vi "PIM Update Test Results.vi"(5 "PIM Test Results":T11={"Measurement Cycles"=0, "Calibration State"=FALSE, "Data"=[], "PIM Test Parameters"={"Stimulus"={"C1 Pwr dBm"=43.0, "C2 Pwr dBm"=43.0, "Power Units"=enum."dBm", "Meas Type"=enum."Time", "C1 Freq MHz"=0.0, "C2 Freq MHz"=0.0, "Swept Freq Step"=0}, "Measure"={"IM Order"=0, "Direction"=0, "Averaging"=2, "ALC ON?"=TRUE, "Peak Hold?"=TRUE, "Peak last N"=0, "Ref Level dBm"=-100.0, "Ref Units"=enum."dBm", "Num Samples"=0, "Sample units"=enum."Sample(s)", "Update Rate (s)"=0.0, "DUT PORT"=enum."Port 1", "Percent (%)"=100}, "Display"={"Power Scale"={"yRange_min"=-160, "yRange_max"=-60}, "xRange_span"=1}}, "Peak IM Level"=0.0, "Instrument String"="", "Instrument Used"={"ixInstrument"=0, "sxInstrumentId"="", "sDriverId"="", "sDriverType"="", "sSerialNumber"="", "tLastCalibration"=timestamp(0 s since 1904-01-01), "tCalibrationDue"=timestamp(0 s since 1904-01-01), "sConfiguration"=""}} {"PIM Test Parameters"."Stimulus"."Swept Freq Step" items=[".2", ".4", "1.0", "2.0"]; "PIM Test Parameters"."Measure"."Averaging" items=["None", "Minimum", "Normal", "High", "Maximum"]; "PIM Test Parameters"."Measure"."Direction" items=["Reverse", "Forward", "Auxiliary"]; "PIM Test Parameters"."Measure"."IM Order" items=["3rd", "5th", "7th", "9th", "11th", "13th", "15th", "17th", "19th", "21st", "23rd", "25th", "27th", "29th", "31st", "33rd"]}, 7 "Increment Cycles?":bool, 9 "PIM Test Parameters":T1={"Stimulus"={"C1 Pwr dBm"=0.0, "C2 Pwr dBm"=0.0, "Power Units"=enum."dBm", "Meas Type"=enum."Time", "C1 Freq MHz"=0.0, "C2 Freq MHz"=0.0, "Swept Freq Step"=0}, "Measure"={"IM Order"=0, "Direction"=0, "Averaging"=1, "ALC ON?"=TRUE, "Peak Hold?"=TRUE, "Peak last N"=1, "Ref Level dBm"=-100.0, "Ref Units"=enum."dBm", "Num Samples"=1, "Sample units"=enum."Sample(s)", "Update Rate (s)"=0.0, "DUT PORT"=enum."Port 1", "Percent (%)"=100}, "Display"={"Power Scale"={"yRange_min"=0, "yRange_max"=0}, "xRange_span"=5}} {"Stimulus"."Swept Freq Step" items=[".2", ".4", "1.0", "2.0"]; "Measure"."Averaging" items=["None", "Minimum", "Normal", "High", "Maximum"]; "Measure"."Direction" items=["Reverse", "Forward", "Auxiliary"]; "Measure"."IM Order" items=["3rd", "5th", "7th", "9th", "11th", "13th", "15th", "17th", "19th", "21st", "23rd", "25th", "27th", "29th", "31st", "33rd"]}, 10 "Passed?":bool, 12 "Start Time":dbl, 13 "Discard Measurement":bool, 14 "Measurement Results":T13 {"IMPower_dBc(s)" format="%.2f"; "TxFreqs" format="%.2f"; "IMFreq(s)" format="%.2f"; "IMPower(s)" format="%.2f"; "TxPower" format="%.2f"}) -> (6 "Updated Test Results":T11={"Measurement Cycles"=0, "Calibration State"=FALSE, "Data"=[], "PIM Test Parameters"={"Stimulus"={"C1 Pwr dBm"=43.0, "C2 Pwr dBm"=43.0, "Power Units"=enum."dBm", "Meas Type"=enum."Time", "C1 Freq MHz"=0.0, "C2 Freq MHz"=0.0, "Swept Freq Step"=0}, "Measure"={"IM Order"=0, "Direction"=0, "Averaging"=2, "ALC ON?"=TRUE, "Peak Hold?"=TRUE, "Peak last N"=0, "Ref Level dBm"=-100.0, "Ref Units"=enum."dBm", "Num Samples"=0, "Sample units"=enum."Sample(s)", "Update Rate (s)"=0.0, "DUT PORT"=enum."Port 1", "Percent (%)"=100}, "Display"={"Power Scale"={"yRange_min"=-160, "yRange_max"=-60}, "xRange_span"=1}}, "Peak IM Level"=0.0, "Instrument String"="", "Instrument Used"={"ixInstrument"=0, "sxInstrumentId"="", "sDriverId"="", "sDriverType"="", "sSerialNumber"="", "tLastCalibration"=timestamp(0 s since 1904-01-01), "tCalibrationDue"=timestamp(0 s since 1904-01-01), "sConfiguration"=""}} {"PIM Test Parameters"."Stimulus"."Swept Freq Step" items=[".2", ".4", "1.0", "2.0"]; "PIM Test Parameters"."Measure"."Averaging" items=["None", "Minimum", "Normal", "High", "Maximum"]; "PIM Test Parameters"."Measure"."Direction" items=["Reverse", "Forward", "Auxiliary"]; "PIM Test Parameters"."Measure"."IM Order" items=["3rd", "5th", "7th", "9th", "11th", "13th", "15th", "17th", "19th", "21st", "23rd", "25th", "27th", "29th", "31st", "33rd"]})   [LabVIEW 2011]
uses:
  TypeDefs/PIM Test Results.ctl
  TypeDefs/PIM Test Parameters.ctl
  TypeDefs/PIM Stimulus Parameters.ctl
  BPIMCore/HW IO/PIM Sweep Step Size.ctl
  TypeDefs/PIM Measurement Parameters.ctl
  BPIMCore/HW IO/IMOrder.ctl
  BPIMCore/HW IO/MeasMode.ctl
  BPIMCore/HW IO/HW Averaging.ctl
  TypeDefs/PIM Meas Units.ctl
  BPIMCore/HW IO/DUTport.ctl
  TypeDefs/PIM Display Parameters.ctl
  typedefs/Instrument Record.ctl
  drivers/PIM/PIM Results.ctl
  TypeDefs/PIM Data Channels.ctl
  Channel Test Status Enumeration.ctl
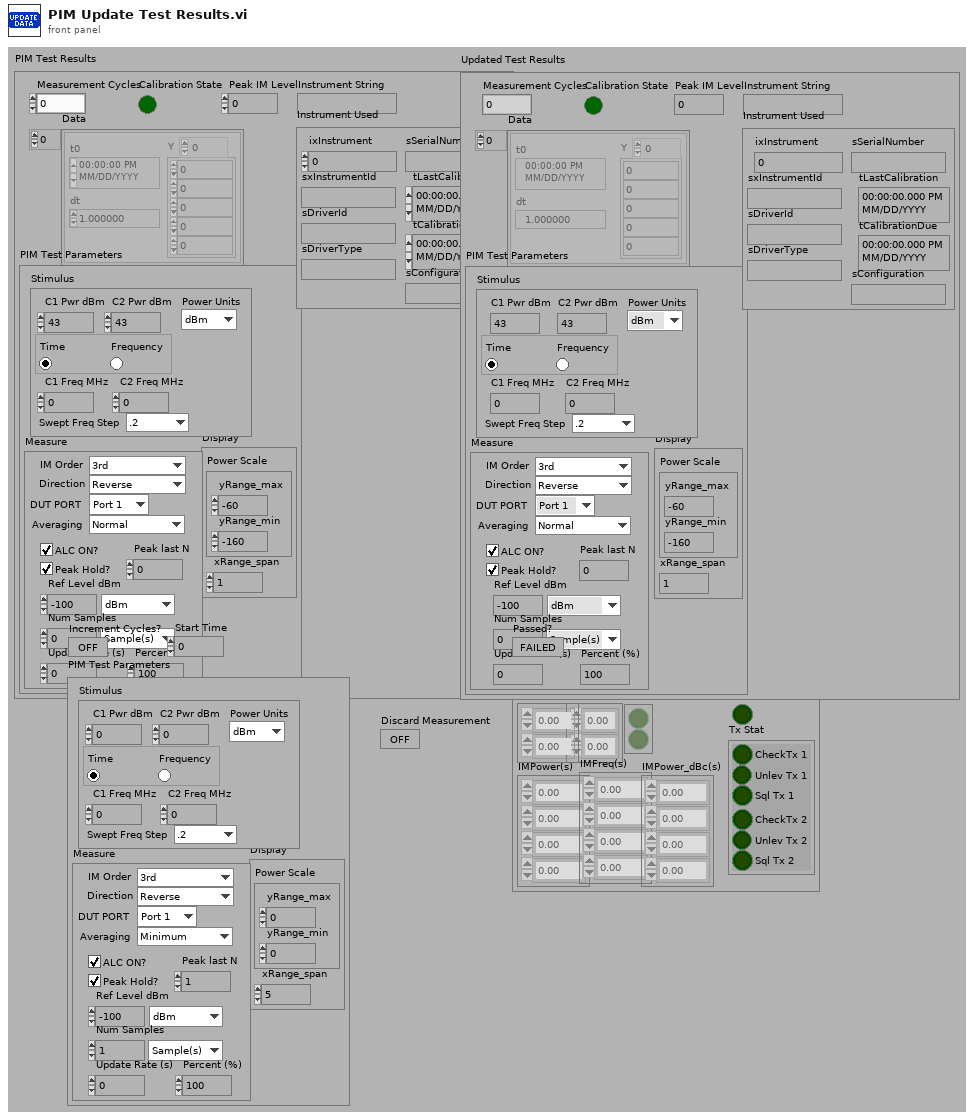
[diagram p1: front panel]
types:
  T1 = typedef "PIM Test Parameters.ctl" = cluster{"Stimulus":T2, "Measure":T4, "Display":T10}
  T2 = typedef "PIM Stimulus Parameters.ctl" = cluster{"C1 Pwr dBm":dbl, "C2 Pwr dBm":dbl, "Power Units":enum16{"dBm", "Watts"}, "Meas Type":enum32{"Time", "Frequency"}, "C1 Freq MHz":dbl, "C2 Freq MHz":dbl, "Swept Freq Step":T3}
  T3 = typedef "PIM Sweep Step Size.ctl" = u16
  T4 = typedef "PIM Measurement Parameters.ctl" = cluster{"IM Order":T5, "Direction":T6, "Averaging":T7, "ALC ON?":bool, "Peak Hold?":bool, "Peak last N":u32, "Ref Level dBm":dbl, "Ref Units":enum16{"dBm", "dBc"}, "Num Samples":u32, "Sample units":T8, "Update Rate (s)":dbl, "DUT PORT":T9, "Percent (%)":u8}
  T5 = typedef "IMOrder.ctl" = u8
  T6 = typedef "MeasMode.ctl" = u16
  T7 = typedef "HW Averaging.ctl" = u16
  T8 = typedef "PIM Meas Units.ctl" = enum16{"Sample(s)", "Second(s)", "Sweep(s)"}
  T9 = typedef "DUTport.ctl" = enum16{"Port 1", "Port 2"}
  T10 = typedef "PIM Display Parameters.ctl" = cluster{"Power Scale":cluster{"yRange_min":i32, "yRange_max":i32}, "xRange_span":u32}
  T11 = typedef "PIM Test Results.ctl" = cluster{"Measurement Cycles":i32, "Calibration State":bool, "Data":waveform(dbl)[], "PIM Test Parameters":T1, "Peak IM Level":dbl, "Instrument String":string, "Instrument Used":T12}
  T12 = typedef "Instrument Record.ctl" = cluster{"ixInstrument":i32, "sxInstrumentId":string, "sDriverId":string, "sDriverType":string, "sSerialNumber":string, "tLastCalibration":timestamp, "tCalibrationDue":timestamp, "sConfiguration":string}
  T13 = typedef "PIM Results.ctl" = cluster{"TxFreqs":dbl[], "TxPower":dbl[], "TxOn":bool[], "IMPower(s)":dbl[], "IMFreq(s)":dbl[], "Tx Stat":cluster{"CheckTx 1":bool, "Unlev Tx 1":bool, "Sql Tx 1":bool, "CheckTx 2":bool, "Unlev Tx 2":bool, "Sql Tx 2":bool}, "IM Overload":bool, "IMPower_dBc(s)":dbl[]}
  T14 = typedef "PIM Data Channels.ctl" = enum16{"Tx1 Frequency", "Tx1 Power", "Tx1 Check Tx", "Tx1 Unleveled", "Tx1 Squelch", "Tx2 Frequency", "Tx2 Power", "Tx2 Check Tx", "Tx2 Unleveled", "Tx2 Squelch", "Elapsed Time", "Ref Limit 1", "Ref Limit 2", "IM Overload", "IM%d Frequency", "IM%d Power 1", "IM%d Power 2"}
  T15 = typedef "Channel Test Status Enumeration.ctl" = enum16{"Fail", "Pass", "Abort", "Error", "Done", "Pass by Sample", "Fail by Sample", "Pass Override", "Fail Override", "Not Tested"}
  T16 = cluster{"CheckTx 1":bool, "Unlev Tx 1":bool, "Sql Tx 1":bool, "CheckTx 2":bool, "Unlev Tx 2":bool, "Sql Tx 2":bool}
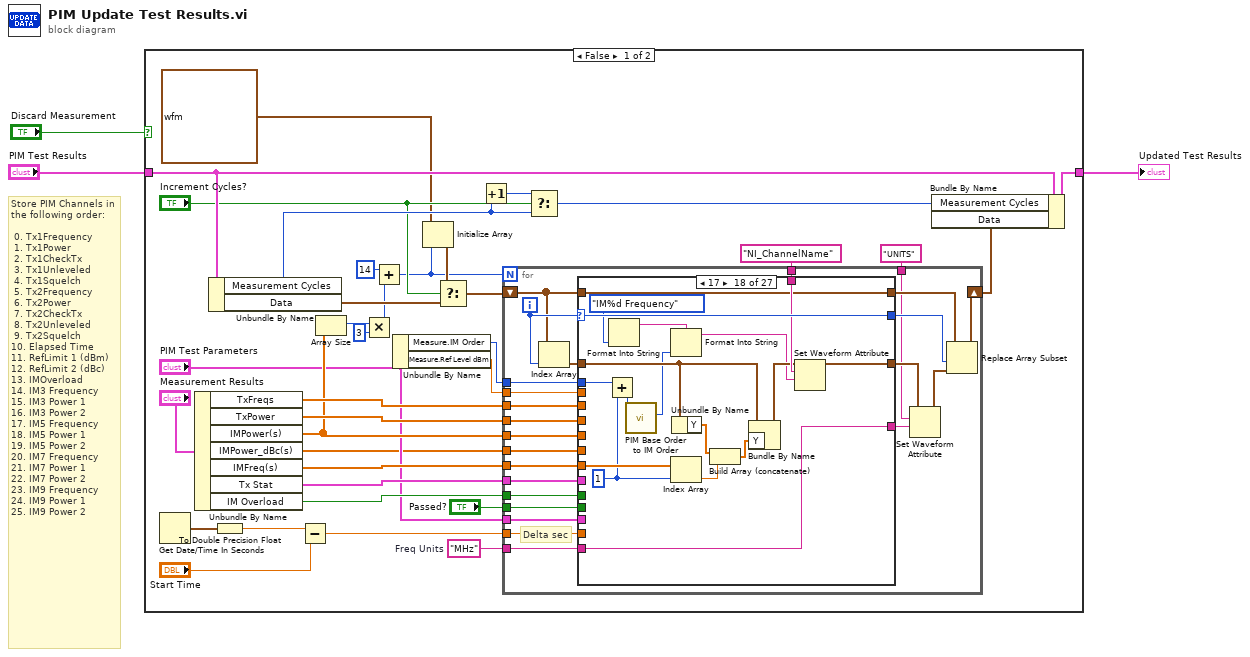
[diagram p0: block diagram]
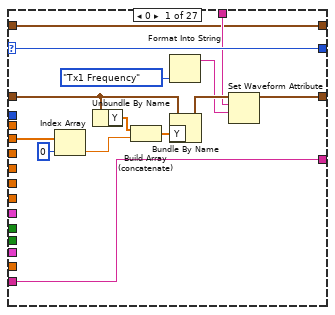
[diagram p2: hidden frame]
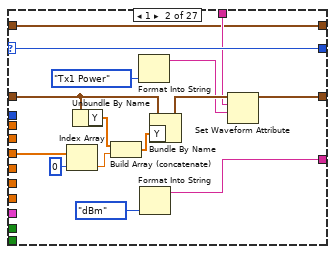
[diagram p3: hidden frame]
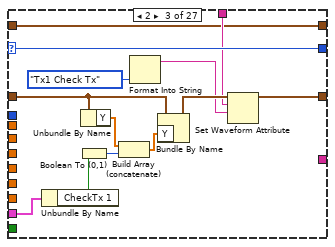
[diagram p4: hidden frame]
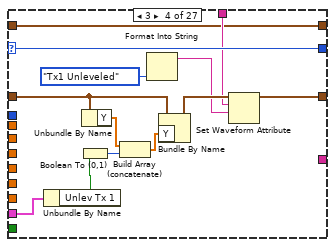
[diagram p5: hidden frame]
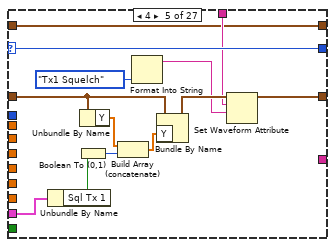
[diagram p6: hidden frame]
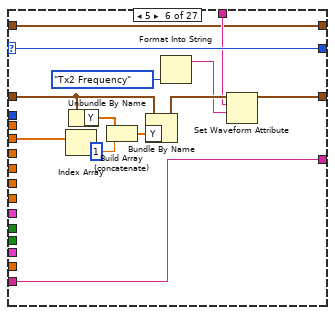
[diagram p7: hidden frame]
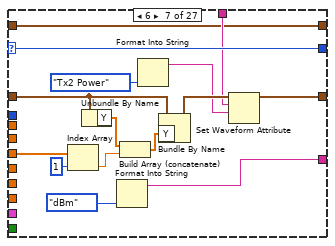
[diagram p8: hidden frame]
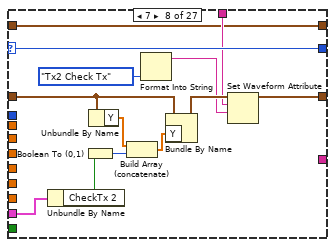
[diagram p9: hidden frame]
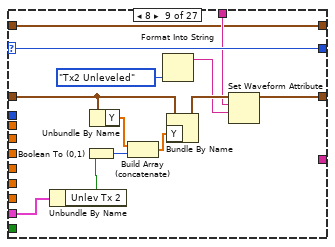
[diagram p10: hidden frame]
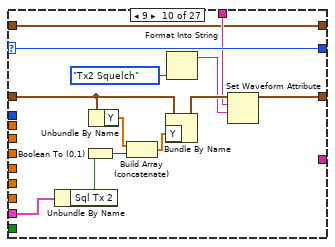
[diagram p11: hidden frame]
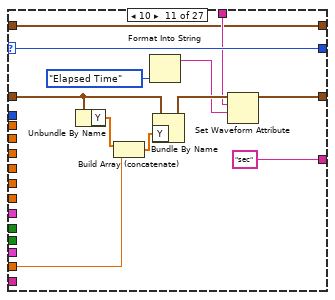
[diagram p12: hidden frame]
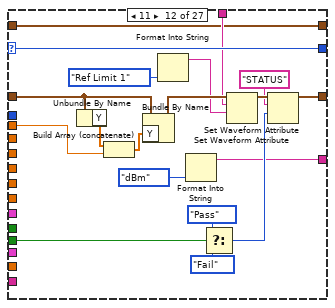
[diagram p13: hidden frame]
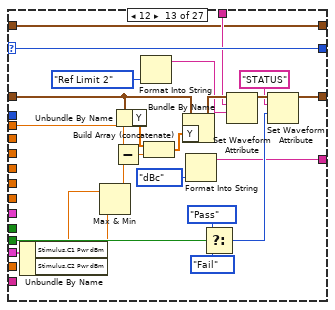
[diagram p14: hidden frame]
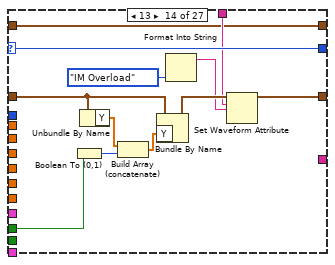
[diagram p15: hidden frame]
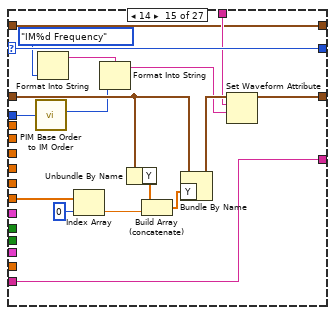
[diagram p16: hidden frame]
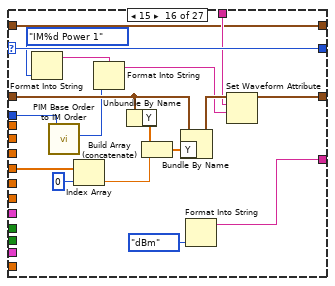
[diagram p17: hidden frame]
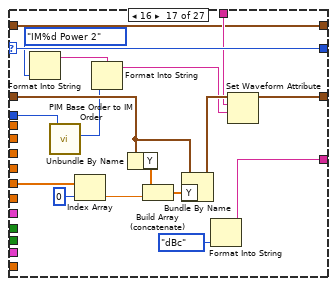
[diagram p18: hidden frame]
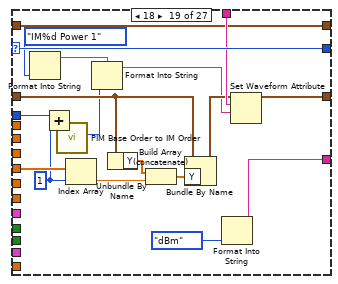
[diagram p19: hidden frame]
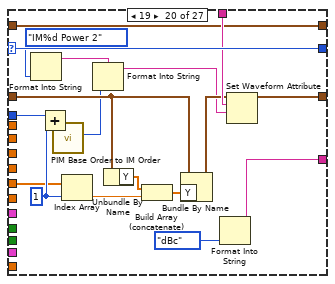
[diagram p20: hidden frame]
diagram:
  # "Store PIM Channels in the following order:\n\n 0. Tx1Frequency\n 1. Tx1Power\n 2. Tx1CheckTx\n 3. Tx1Unleveled\n 4. Tx1Squelch\n 5. Tx2Frequency\n 6. Tx2Power\n 7. Tx2CheckTx\n 8. Tx2Unleveled\n 9. Tx2Squelch\n10. Elapsed Time\n11. RefLimit 1 (dBm)\n12. RefLimit 2 (dBc)\n13. IMOverload\n14. IM3 Frequency\n15. IM3 Power 1\n16. IM3 Power 2\n17. IM5 Frequency\n18. IM5 Power 1\n19. IM5 Power 2\n20. IM7 Frequency\n21. IM7 Power 1\n22. IM7 Power 2\n23. IM9 Frequency\n24. IM9 Power 1\n25. IM9 Power 2"
  n1 = case shown="False" "Discard Measurement" {
    tunnel: "PIM Test Results" -> [w38 w491]
    tunnel: [w37 w491] -> w2
    frame False {
      w10 = "MHz"  # Freq Units
      n2 = Get Date/Time In Seconds() -> (seconds since 1Jan1904=w28:timestamp)
      n3 = Unbundle By Name("Measurement Results") -> ("TxFreqs"=w33:dbl[], "TxPower"=w32:dbl[], "IMPower(s)"=w16:dbl[], "IMPower_dBc(s)"=w5:dbl[], "IMFreq(s)"=w31:dbl[], "Tx Stat"=w30:T16, "IM Overload"=w29:bool)
      n4 = Unbundle By Name(w38) -> ("Measurement Cycles"=w36:i32, "Data"=w22:waveform(dbl)[])
      n5 = To Double Precision Float(number=w28) -> (double precision float=w27:dbl)
      n6 = Subtract(x=w27, y="Start Time") -> (x-y=w25:dbl)
      n7 = Array Size(array=w16) -> (size(s)=w13:i32)
      n8 = Multiply(x=w13, y=3) -> (x*y=w11:i32)
      n9 = Add(x=14, y=w11) -> (x+y=w14:i32)
      n10 = Unbundle By Name("PIM Test Parameters") -> ("Measure.IM Order"=w6:T5, "Measure.Ref Level dBm"=w17:dbl)
      n11 = Initialize Array(waveform(dbl) {"t0"=timestamp(0 s since 1904-01-01), "dt"=1.0, "Y"=[]} ("waveform"), w14) -> (w18:waveform(dbl)[])
      n12 = Select(t=w18, s="Increment Cycles?", f=w22) -> (s? t:f=w21:waveform(dbl)[])
      n13 = Increment(x=w36) -> (x+1=w35:i32)
      n14 = for {
        N: w14 -> [_]
        tunnel: w33 -> [w62]
        tunnel: w32 -> [w61]
        tunnel: w16 -> [w60]
        tunnel: w31 -> [w59]
        tunnel: w30 -> [w58]
        tunnel: w29 -> [w57]
        shift-right: [w54] -> w24
        shift-left: w21 -> [w47]
        tunnel: w25 -> [w52]
        tunnel: "NI_ChannelName" -> [w51]
        tunnel: "Passed?" -> [w50]
        tunnel: w17 -> [w49]
        tunnel: w6 -> [w48]
        tunnel: w10 -> [w45]
        tunnel: "UNITS" -> [w42]
        tunnel: "PIM Test Parameters" -> [w40]
        tunnel: w5 -> [w39]
        i -> [w55]
        # "Delta sec"
        n15 = Index Array(array=w47, index=w55) -> (element=w56:waveform(dbl))
        n16 = case shown="17" w55 {
          selector: w55 -> [w69 w83 w99 w112 w125 w137 w152 w167 w180 w193 w205 w225 w249 w260 w277 w295 w313 w334 w353 w372 w392 w411 w430 w448 w467 w486 w489]
          tunnel: w62 -> [w76 _ _ _ _ w136 _ _ _ _ _ _ _ _ _ _ _ _ _ _ _ _ _ _ _ _ _]
          tunnel: w61 -> [_ w84 _ _ _ _ w151 _ _ _ _ _ _ _ _ _ _ _ _ _ _ _ _ _ _ _ _]
          tunnel: w60 -> [_ _ _ _ _ _ _ _ _ _ _ _ _ _ _ w292 _ _ w351 _ _ w406 _ _ w462 _ _]
          tunnel: w59 -> [_ _ _ _ _ _ _ _ _ _ _ _ _ _ w276 _ _ w331 _ _ w387 _ _ w444 _ _ _]
          tunnel: w58 -> [_ _ w98 w111 w124 _ _ w166 w179 w192 _ _ _ _ _ _ _ _ _ _ _ _ _ _ _ _ _]
          tunnel: w57 -> [_ _ _ _ _ _ _ _ _ _ _ _ _ w259 _ _ _ _ _ _ _ _ _ _ _ _ _]
          tunnel: w56 -> [w71 w87 w102 w115 w128 w140 w155 w170 w183 w196 w208 w227 w251 w263 w280 w298 w316 w336 w355 w374 w391 w409 w428 w445 w464 w483 w490]
          tunnel: [w66 w85 w100 w113 w126 w138 w153 w168 w181 w194 w206 w222 w246 w261 w278 w296 w314 w335 w354 w373 w390 w410 w429 w446 w465 w484 w490] -> w43
          tunnel: [w69 w83 w99 w112 w125 w137 w152 w167 w180 w193 w205 w225 w249 w260 w277 w295 w313 w334 w353 w372 w392 w411 w430 w448 w467 w486 w489] -> w53
          tunnel: w52 -> [_ _ _ _ _ _ _ _ _ _ w204 _ _ _ _ _ _ _ _ _ _ _ _ _ _ _ _]
          tunnel: w51 -> [w68 w82 w95 w108 w121 w135 w150 w163 w176 w189 w203 w224 w248 w257 w274 w291 w310 w333 w352 w371 w389 w408 w427 w447 w466 w485 _]
          tunnel: w50 -> [_ _ _ _ _ _ _ _ _ _ _ w218 w242 _ _ _ _ _ _ _ _ _ _ _ _ _ _]
          tunnel: w49 -> [_ _ _ _ _ _ _ _ _ _ _ w216 w236 _ _ _ _ _ _ _ _ _ _ _ _ _ _]
          tunnel: w48 -> [_ _ _ _ _ _ _ _ _ _ _ _ _ _ w273 w290 w309 w332 w349 w369 w386 w407 w426 w442 w463 w482 _]
          tunnel: w47 -> [w67 w81 w94 w107 w120 w134 w149 w162 w175 w188 w202 w215 w240 w256 w271 w289 w308 w329 w348 w368 w385 w404 w424 w441 w460 w480 w488]
          tunnel: [w67 w81 w94 w107 w120 w134 w149 w162 w175 w188 w202 w215 w240 w256 w271 w289 w308 w329 w348 w368 w385 w404 w424 w441 w460 w480 w487] -> w46
          tunnel: w45 -> [w65 _ _ _ _ w133 _ _ _ _ _ _ _ _ w270 _ _ w323 _ _ w379 _ _ w435 _ _ _]
          tunnel: [w65 w79 _ _ _ w133 w147 _ _ _ "sec" w214 w239 _ w270 w288 w307 w323 w342 w362 w379 w398 w418 w435 w454 w474 _] -> w41
          tunnel: w40 -> [_ _ _ _ _ _ _ _ _ _ _ _ w235 _ _ _ _ _ _ _ _ _ _ _ _ _ _]
          tunnel: w39 -> [_ _ _ _ _ _ _ _ _ _ _ _ _ _ _ _ w305 _ _ w360 _ _ w416 _ _ w472 _]
          frame 0 {
            n17 = Index Array(array=w76, index=0) -> (element=w73:dbl)
            n18 = Unbundle By Name(w71) -> ("Y"=w74:dbl[])
            n19 = Build Array (concatenate)(w74, w73) -> (w72:dbl[])
            n20 = Format Into String(PIM_Data_Channels."Tx1 Frequency" ("Enum")) -> (resulting string=w63:string)  [unwired: 3 in, 1 out]
            n21 = Bundle By Name(cluster=w71, "Y"=w72) -> (w70:waveform(dbl))
            n22 = Set Waveform Attribute(5:w63, 6:w68, 7:w70) -> (3:w66:waveform(dbl))  [unwired: 1 in, 2 out]
          }
          frame 1 {
            n23 = Index Array(array=w84, index=0) -> (element=w89:dbl)
            n24 = Unbundle By Name(w87) -> ("Y"=w90:dbl[])
            n25 = Build Array (concatenate)(w90, w89) -> (w88:dbl[])
            n26 = Format Into String(PIM_Data_Channels."Tx1 Power" ("Enum")) -> (resulting string=w77:string)  [unwired: 3 in, 1 out]
            n27 = Format Into String(enum16{"dBm", "Watts"}."dBm" ("PIM Test Stimulus.Power Units")) -> (resulting string=w79:string)  [unwired: 3 in, 1 out]
            n28 = Bundle By Name(cluster=w87, "Y"=w88) -> (w86:waveform(dbl))
            n29 = Set Waveform Attribute(5:w77, 6:w82, 7:w86) -> (3:w85:waveform(dbl))  [unwired: 1 in, 2 out]
          }
          frame 2 {
            n30 = Unbundle By Name(w98) -> ("CheckTx 1"=w97:bool)
            n31 = Boolean To (0,1)(Boolean=w97) -> (0, 1=w96:i16)
            n32 = Unbundle By Name(w102) -> ("Y"=w104:dbl[])
            n33 = Build Array (concatenate)(w104, w96) -> (w103:dbl[])
            n34 = Format Into String(PIM_Data_Channels."Tx1 Check Tx" ("Enum")) -> (resulting string=w92:string)  [unwired: 3 in, 1 out]
            n35 = Bundle By Name(cluster=w102, "Y"=w103) -> (w101:waveform(dbl))
            n36 = Set Waveform Attribute(5:w92, 6:w95, 7:w101) -> (3:w100:waveform(dbl))  [unwired: 1 in, 2 out]
          }
          frame 3 {
            n37 = Unbundle By Name(w111) -> ("Unlev Tx 1"=w110:bool)
            n38 = Boolean To (0,1)(Boolean=w110) -> (0, 1=w109:i16)
            n39 = Unbundle By Name(w115) -> ("Y"=w117:dbl[])
            n40 = Build Array (concatenate)(w117, w109) -> (w116:dbl[])
            n41 = Format Into String(PIM_Data_Channels."Tx1 Unleveled" ("Enum")) -> (resulting string=w105:string)  [unwired: 3 in, 1 out]
            n42 = Bundle By Name(cluster=w115, "Y"=w116) -> (w114:waveform(dbl))
            n43 = Set Waveform Attribute(5:w105, 6:w108, 7:w114) -> (3:w113:waveform(dbl))  [unwired: 1 in, 2 out]
          }
          frame 4 {
            n44 = Unbundle By Name(w124) -> ("Sql Tx 1"=w123:bool)
            n45 = Boolean To (0,1)(Boolean=w123) -> (0, 1=w122:i16)
            n46 = Unbundle By Name(w128) -> ("Y"=w130:dbl[])
            n47 = Build Array (concatenate)(w130, w122) -> (w129:dbl[])
            n48 = Format Into String(PIM_Data_Channels."Tx1 Squelch" ("Enum")) -> (resulting string=w118:string)  [unwired: 3 in, 1 out]
            n49 = Bundle By Name(cluster=w128, "Y"=w129) -> (w127:waveform(dbl))
            n50 = Set Waveform Attribute(5:w118, 6:w121, 7:w127) -> (3:w126:waveform(dbl))  [unwired: 1 in, 2 out]
          }
          frame 5 {
            n51 = Index Array(array=w136, index=1) -> (element=w142:dbl)
            n52 = Unbundle By Name(w140) -> ("Y"=w143:dbl[])
            n53 = Build Array (concatenate)(w143, w142) -> (w141:dbl[])
            n54 = Bundle By Name(cluster=w140, "Y"=w141) -> (w139:waveform(dbl))
            n55 = Format Into String(PIM_Data_Channels."Tx2 Frequency" ("Enum")) -> (resulting string=w131:string)  [unwired: 3 in, 1 out]
            n56 = Set Waveform Attribute(5:w131, 6:w135, 7:w139) -> (3:w138:waveform(dbl))  [unwired: 1 in, 2 out]
          }
          frame 6 {
            n57 = Index Array(array=w151, index=1) -> (element=w157:dbl)
            n58 = Unbundle By Name(w155) -> ("Y"=w158:dbl[])
            n59 = Format Into String(enum16{"dBm", "Watts"}."dBm" ("PIM Test Stimulus.Power Units")) -> (resulting string=w147:string)  [unwired: 3 in, 1 out]
            n60 = Build Array (concatenate)(w158, w157) -> (w156:dbl[])
            n61 = Format Into String(PIM_Data_Channels."Tx2 Power" ("Enum")) -> (resulting string=w145:string)  [unwired: 3 in, 1 out]
            n62 = Bundle By Name(cluster=w155, "Y"=w156) -> (w154:waveform(dbl))
            n63 = Set Waveform Attribute(5:w145, 6:w150, 7:w154) -> (3:w153:waveform(dbl))  [unwired: 1 in, 2 out]
          }
          frame 7 {
            n64 = Unbundle By Name(w166) -> ("CheckTx 2"=w165:bool)
            n65 = Boolean To (0,1)(Boolean=w165) -> (0, 1=w164:i16)
            n66 = Unbundle By Name(w170) -> ("Y"=w172:dbl[])
            n67 = Build Array (concatenate)(w172, w164) -> (w171:dbl[])
            n68 = Format Into String(PIM_Data_Channels."Tx2 Check Tx" ("Enum")) -> (resulting string=w160:string)  [unwired: 3 in, 1 out]
            n69 = Bundle By Name(cluster=w170, "Y"=w171) -> (w169:waveform(dbl))
            n70 = Set Waveform Attribute(5:w160, 6:w163, 7:w169) -> (3:w168:waveform(dbl))  [unwired: 1 in, 2 out]
          }
          frame 8 {
            n71 = Unbundle By Name(w179) -> ("Unlev Tx 2"=w178:bool)
            n72 = Boolean To (0,1)(Boolean=w178) -> (0, 1=w177:i16)
            n73 = Unbundle By Name(w183) -> ("Y"=w185:dbl[])
            n74 = Build Array (concatenate)(w185, w177) -> (w184:dbl[])
            n75 = Format Into String(PIM_Data_Channels."Tx2 Unleveled" ("Enum")) -> (resulting string=w173:string)  [unwired: 3 in, 1 out]
            n76 = Bundle By Name(cluster=w183, "Y"=w184) -> (w182:waveform(dbl))
            n77 = Set Waveform Attribute(5:w173, 6:w176, 7:w182) -> (3:w181:waveform(dbl))  [unwired: 1 in, 2 out]
          }
          frame 9 {
            n78 = Unbundle By Name(w192) -> ("Sql Tx 2"=w191:bool)
            n79 = Boolean To (0,1)(Boolean=w191) -> (0, 1=w190:i16)
            n80 = Unbundle By Name(w196) -> ("Y"=w198:dbl[])
            n81 = Build Array (concatenate)(w198, w190) -> (w197:dbl[])
            n82 = Bundle By Name(cluster=w196, "Y"=w197) -> (w195:waveform(dbl))
            n83 = Format Into String(PIM_Data_Channels."Tx2 Squelch" ("Enum")) -> (resulting string=w186:string)  [unwired: 3 in, 1 out]
            n84 = Set Waveform Attribute(5:w186, 6:w189, 7:w195) -> (3:w194:waveform(dbl))  [unwired: 1 in, 2 out]
          }
          frame 10 {
            n85 = Unbundle By Name(w208) -> ("Y"=w210:dbl[])
            n86 = Build Array (concatenate)(w210, w204) -> (w209:dbl[])
            n87 = Format Into String(PIM_Data_Channels."Elapsed Time" ("Enum")) -> (resulting string=w199:string)  [unwired: 3 in, 1 out]
            n88 = Bundle By Name(cluster=w208, "Y"=w209) -> (w207:waveform(dbl))
            n89 = Set Waveform Attribute(5:w199, 6:w203, 7:w207) -> (3:w206:waveform(dbl))  [unwired: 1 in, 2 out]
          }
          frame 11 {
            n90 = Unbundle By Name(w227) -> ("Y"=w229:dbl[])
            n91 = Build Array (concatenate)(w229, w216) -> (w228:dbl[])
            n92 = Bundle By Name(cluster=w227, "Y"=w228) -> (w226:waveform(dbl))
            n93 = Format Into String(PIM_Data_Channels."Ref Limit 1" ("Enum")) -> (resulting string=w211:string)  [unwired: 3 in, 1 out]
            n94 = Format Into String(enum16{"dBm", "dBc"}."dBm" ("Measure.Ref Units")) -> (resulting string=w214:string)  [unwired: 3 in, 1 out]
            n95 = Select(t=Channel_Test_Status_Enumeration."Pass" ("Channel Status Enumeration"), s=w218, f=Channel_Test_Status_Enumeration."Fail" ("Channel Status Enumeration")) -> (s? t:f=w217:T15)
            n96 = Set Waveform Attribute(5:w211, 6:w224, 7:w226) -> (3:w223:waveform(dbl))  [unwired: 1 in, 2 out]
            n97 = Set Waveform Attribute(5:w217, 6:"STATUS", 7:w223) -> (3:w222:waveform(dbl))  [unwired: 1 in, 2 out]
          }
          frame 12 {
            n98 = Unbundle By Name(w235) -> ("Stimulus.C1 Pwr dBm"=w234:dbl, "Stimulus.C2 Pwr dBm"=w233:dbl)
            n99 = Max & Min(x=w234, y=w233) -> (max(x,y)=w237:dbl)  [unwired: 1 out]
            n100 = Subtract(x=w236, y=w237) -> (x-y=w232:dbl)
            n101 = Unbundle By Name(w251) -> ("Y"=w253:dbl[])
            n102 = Format Into String(PIM_Data_Channels."Ref Limit 2" ("Enum")) -> (resulting string=w230:string)  [unwired: 3 in, 1 out]
            n103 = Build Array (concatenate)(w253, w232) -> (w252:dbl[])
            n104 = Bundle By Name(cluster=w251, "Y"=w252) -> (w250:waveform(dbl))
            n105 = Format Into String(enum16{"dBm", "dBc"}."dBc" ("Measure.Ref Units")) -> (resulting string=w239:string)  [unwired: 3 in, 1 out]
            n106 = Select(t=Channel_Test_Status_Enumeration."Pass" ("Channel Status Enumeration"), s=w242, f=Channel_Test_Status_Enumeration."Fail" ("Channel Status Enumeration")) -> (s? t:f=w241:T15)
            n107 = Set Waveform Attribute(5:w230, 6:w248, 7:w250) -> (3:w247:waveform(dbl))  [unwired: 1 in, 2 out]
            n108 = Set Waveform Attribute(5:w241, 6:"STATUS", 7:w247) -> (3:w246:waveform(dbl))  [unwired: 1 in, 2 out]
          }
          frame 13 {
            n109 = Boolean To (0,1)(Boolean=w259) -> (0, 1=w258:i16)
            n110 = Unbundle By Name(w263) -> ("Y"=w265:dbl[])
            n111 = Build Array (concatenate)(w265, w258) -> (w264:dbl[])
            n112 = Bundle By Name(cluster=w263, "Y"=w264) -> (w262:waveform(dbl))
            n113 = Format Into String(PIM_Data_Channels."IM Overload" ("Enum")) -> (resulting string=w254:string)  [unwired: 3 in, 1 out]
            n114 = Set Waveform Attribute(5:w254, 6:w257, 7:w262) -> (3:w261:waveform(dbl))  [unwired: 1 in, 2 out]
          }
          frame 14 {
            n115 = call "PIM Base Order to IM Order.vi"("Base Order (0)"=w273) -> ("IM Order"=w266:u8)  [unwired: 5 out]
            n116 = Format Into String(PIM_Data_Channels."IM%d Frequency" ("Enum")) -> (resulting string=w268:string)  [unwired: 3 in, 1 out]
            n117 = Index Array(array=w276, index=0) -> (element=w275:dbl)
            n118 = Format Into String(format string=w268, w266) -> (resulting string=w267:string)  [unwired: 2 in, 1 out]
            n119 = Unbundle By Name(w280) -> ("Y"=w282:dbl[])
            n120 = Build Array (concatenate)(w282, w275) -> (w281:dbl[])
            n121 = Bundle By Name(cluster=w280, "Y"=w281) -> (w279:waveform(dbl))
            n122 = Set Waveform Attribute(5:w267, 6:w274, 7:w279) -> (3:w278:waveform(dbl))  [unwired: 1 in, 2 out]
          }
          frame 15 {
            n123 = Format Into String(PIM_Data_Channels."IM%d Power 1" ("Enum")) -> (resulting string=w286:string)  [unwired: 3 in, 1 out]
            n124 = call "PIM Base Order to IM Order.vi"("Base Order (0)"=w290) -> ("IM Order"=w283:u8)  [unwired: 5 out]
            n125 = Index Array(array=w292, index=0) -> (element=w293:dbl)
            n126 = Format Into String(format string=w286, w283) -> (resulting string=w284:string)  [unwired: 2 in, 1 out]
            n127 = Unbundle By Name(w298) -> ("Y"=w300:dbl[])
            n128 = Build Array (concatenate)(w300, w293) -> (w299:dbl[])
            n129 = Bundle By Name(cluster=w298, "Y"=w299) -> (w297:waveform(dbl))
            n130 = Format Into String(enum16{"dBm", "dBc"}."dBm" ("Measure.Ref Units")) -> (resulting string=w288:string)  [unwired: 3 in, 1 out]
            n131 = Set Waveform Attribute(5:w284, 6:w291, 7:w297) -> (3:w296:waveform(dbl))  [unwired: 1 in, 2 out]
          }
          frame 16 {
            n132 = Format Into String(PIM_Data_Channels."IM%d Power 2" ("Enum")) -> (resulting string=w303:string)  [unwired: 3 in, 1 out]
            n133 = call "PIM Base Order to IM Order.vi"("Base Order (0)"=w309) -> ("IM Order"=w301:u8)  [unwired: 5 out]
            n134 = Index Array(array=w305, index=0) -> (element=w311:dbl)
            n135 = Format Into String(format string=w303, w301) -> (resulting string=w302:string)  [unwired: 2 in, 1 out]
            n136 = Unbundle By Name(w316) -> ("Y"=w318:dbl[])
            n137 = Build Array (concatenate)(w318, w311) -> (w317:dbl[])
            n138 = Bundle By Name(cluster=w316, "Y"=w317) -> (w315:waveform(dbl))
            n139 = Format Into String(enum16{"dBm", "dBc"}."dBc" ("Measure.Ref Units")) -> (resulting string=w307:string)  [unwired: 3 in, 1 out]
            n140 = Set Waveform Attribute(5:w302, 6:w310, 7:w315) -> (3:w314:waveform(dbl))  [unwired: 1 in, 2 out]
          }
          frame 17 {
            w330 = 1 ("index")
            n141 = Add(x=w332, y=w330) -> (x+y=w324:i32)
            n142 = Format Into String(PIM_Data_Channels."IM%d Frequency" ("Enum")) -> (resulting string=w321:string)  [unwired: 3 in, 1 out]
            n143 = call "PIM Base Order to IM Order.vi"("Base Order (0)"=w324) -> ("IM Order"=w319:u8)  [unwired: 5 out]
            n144 = Format Into String(format string=w321, w319) -> (resulting string=w320:string)  [unwired: 2 in, 1 out]
            n145 = Index Array(array=w331, index=w330) -> (element=w325:dbl)
            n146 = Unbundle By Name(w336) -> ("Y"=w328:dbl[])
            n147 = Build Array (concatenate)(w328, w325) -> (w327:dbl[])
            n148 = Bundle By Name(cluster=w336, "Y"=w327) -> (w326:waveform(dbl))
            n149 = Set Waveform Attribute(5:w320, 6:w333, 7:w326) -> (3:w335:waveform(dbl))  [unwired: 1 in, 2 out]
          }
          frame 18 {
            w350 = 1 ("index")
            n150 = Format Into String(PIM_Data_Channels."IM%d Power 1" ("Enum")) -> (resulting string=w340:string)  [unwired: 3 in, 1 out]
            n151 = Add(x=w349, y=w350) -> (x+y=w343:i32)
            n152 = call "PIM Base Order to IM Order.vi"("Base Order (0)"=w343) -> ("IM Order"=w337:u8)  [unwired: 5 out]
            n153 = Index Array(array=w351, index=w350) -> (element=w344:dbl)
            n154 = Format Into String(format string=w340, w337) -> (resulting string=w338:string)  [unwired: 2 in, 1 out]
            n155 = Unbundle By Name(w355) -> ("Y"=w347:dbl[])
            n156 = Build Array (concatenate)(w347, w344) -> (w346:dbl[])
            n157 = Bundle By Name(cluster=w355, "Y"=w346) -> (w345:waveform(dbl))
            n158 = Format Into String(enum16{"dBm", "dBc"}."dBm" ("Measure.Ref Units")) -> (resulting string=w342:string)  [unwired: 3 in, 1 out]
            n159 = Set Waveform Attribute(5:w338, 6:w352, 7:w345) -> (3:w354:waveform(dbl))  [unwired: 1 in, 2 out]
          }
          frame 19 {
            w370 = 1 ("index")
            n160 = Format Into String(PIM_Data_Channels."IM%d Power 2" ("Enum")) -> (resulting string=w358:string)  [unwired: 3 in, 1 out]
            n161 = Add(x=w369, y=w370) -> (x+y=w363:i32)
            n162 = call "PIM Base Order to IM Order.vi"("Base Order (0)"=w363) -> ("IM Order"=w356:u8)  [unwired: 5 out]
            n163 = Index Array(array=w360, index=w370) -> (element=w364:dbl)
            n164 = Format Into String(format string=w358, w356) -> (resulting string=w357:string)  [unwired: 2 in, 1 out]
            n165 = Unbundle By Name(w374) -> ("Y"=w367:dbl[])
            n166 = Build Array (concatenate)(w367, w364) -> (w366:dbl[])
            n167 = Bundle By Name(cluster=w374, "Y"=w366) -> (w365:waveform(dbl))
            n168 = Format Into String(enum16{"dBm", "dBc"}."dBc" ("Measure.Ref Units")) -> (resulting string=w362:string)  [unwired: 3 in, 1 out]
            n169 = Set Waveform Attribute(5:w357, 6:w371, 7:w365) -> (3:w373:waveform(dbl))  [unwired: 1 in, 2 out]
          }
          frame 20 {
            w388 = 2 ("index")
            n170 = Add(x=w386, y=w388) -> (x+y=w380:i32)
            n171 = Format Into String(PIM_Data_Channels."IM%d Frequency" ("Enum")) -> (resulting string=w377:string)  [unwired: 3 in, 1 out]
            n172 = call "PIM Base Order to IM Order.vi"("Base Order (0)"=w380) -> ("IM Order"=w375:u8)  [unwired: 5 out]
            n173 = Format Into String(format string=w377, w375) -> (resulting string=w376:string)  [unwired: 2 in, 1 out]
            n174 = Index Array(array=w387, index=w388) -> (element=w381:dbl)
            n175 = Unbundle By Name(w391) -> ("Y"=w384:dbl[])
            n176 = Build Array (concatenate)(w384, w381) -> (w383:dbl[])
            n177 = Bundle By Name(cluster=w391, "Y"=w383) -> (w382:waveform(dbl))
            n178 = Set Waveform Attribute(5:w376, 6:w389, 7:w382) -> (3:w390:waveform(dbl))  [unwired: 1 in, 2 out]
          }
          frame 21 {
            w405 = 2 ("index")
            n179 = Format Into String(PIM_Data_Channels."IM%d Power 1" ("Enum")) -> (resulting string=w396:string)  [unwired: 3 in, 1 out]
            n180 = Add(x=w407, y=w405) -> (x+y=w399:i32)
            n181 = call "PIM Base Order to IM Order.vi"("Base Order (0)"=w399) -> ("IM Order"=w393:u8)  [unwired: 5 out]
            n182 = Index Array(array=w406, index=w405) -> (element=w400:dbl)
            n183 = Format Into String(format string=w396, w393) -> (resulting string=w394:string)  [unwired: 2 in, 1 out]
            n184 = Unbundle By Name(w409) -> ("Y"=w403:dbl[])
            n185 = Build Array (concatenate)(w403, w400) -> (w402:dbl[])
            n186 = Bundle By Name(cluster=w409, "Y"=w402) -> (w401:waveform(dbl))
            n187 = Format Into String(enum16{"dBm", "dBc"}."dBm" ("Measure.Ref Units")) -> (resulting string=w398:string)  [unwired: 3 in, 1 out]
            n188 = Set Waveform Attribute(5:w394, 6:w408, 7:w401) -> (3:w410:waveform(dbl))  [unwired: 1 in, 2 out]
          }
          frame 22 {
            w425 = 2 ("index")
            n189 = Format Into String(PIM_Data_Channels."IM%d Power 2" ("Enum")) -> (resulting string=w414:string)  [unwired: 3 in, 1 out]
            n190 = Add(x=w426, y=w425) -> (x+y=w419:i32)
            n191 = call "PIM Base Order to IM Order.vi"("Base Order (0)"=w419) -> ("IM Order"=w412:u8)  [unwired: 5 out]
            n192 = Index Array(array=w416, index=w425) -> (element=w420:dbl)
            n193 = Format Into String(format string=w414, w412) -> (resulting string=w413:string)  [unwired: 2 in, 1 out]
            n194 = Unbundle By Name(w428) -> ("Y"=w423:dbl[])
            n195 = Build Array (concatenate)(w423, w420) -> (w422:dbl[])
            n196 = Bundle By Name(cluster=w428, "Y"=w422) -> (w421:waveform(dbl))
            n197 = Format Into String(enum16{"dBm", "dBc"}."dBc" ("Measure.Ref Units")) -> (resulting string=w418:string)  [unwired: 3 in, 1 out]
            n198 = Set Waveform Attribute(5:w413, 6:w427, 7:w421) -> (3:w429:waveform(dbl))  [unwired: 1 in, 2 out]
          }
          frame 23 {
            w443 = 3 ("index")
            n199 = Add(x=w442, y=w443) -> (x+y=w436:i32)
            n200 = Format Into String(PIM_Data_Channels."IM%d Frequency" ("Enum")) -> (resulting string=w433:string)  [unwired: 3 in, 1 out]
            n201 = call "PIM Base Order to IM Order.vi"("Base Order (0)"=w436) -> ("IM Order"=w431:u8)  [unwired: 5 out]
            n202 = Index Array(array=w444, index=w443) -> (element=w437:dbl)
            n203 = Format Into String(format string=w433, w431) -> (resulting string=w432:string)  [unwired: 2 in, 1 out]
            n204 = Unbundle By Name(w445) -> ("Y"=w440:dbl[])
            n205 = Build Array (concatenate)(w440, w437) -> (w439:dbl[])
            n206 = Bundle By Name(cluster=w445, "Y"=w439) -> (w438:waveform(dbl))
            n207 = Set Waveform Attribute(5:w432, 6:w447, 7:w438) -> (3:w446:waveform(dbl))  [unwired: 1 in, 2 out]
          }
          frame 24 {
            w461 = 3 ("index")
            n208 = Format Into String(PIM_Data_Channels."IM%d Power 1" ("Enum")) -> (resulting string=w452:string)  [unwired: 3 in, 1 out]
            n209 = Add(x=w463, y=w461) -> (x+y=w455:i32)
            n210 = call "PIM Base Order to IM Order.vi"("Base Order (0)"=w455) -> ("IM Order"=w449:u8)  [unwired: 5 out]
            n211 = Index Array(array=w462, index=w461) -> (element=w456:dbl)
            n212 = Format Into String(format string=w452, w449) -> (resulting string=w450:string)  [unwired: 2 in, 1 out]
            n213 = Unbundle By Name(w464) -> ("Y"=w459:dbl[])
            n214 = Build Array (concatenate)(w459, w456) -> (w458:dbl[])
            n215 = Bundle By Name(cluster=w464, "Y"=w458) -> (w457:waveform(dbl))
            n216 = Set Waveform Attribute(5:w450, 6:w466, 7:w457) -> (3:w465:waveform(dbl))  [unwired: 1 in, 2 out]
            n217 = Format Into String(enum16{"dBm", "dBc"}."dBm" ("Measure.Ref Units")) -> (resulting string=w454:string)  [unwired: 3 in, 1 out]
          }
          frame 25 {
            w481 = 3 ("index")
            n218 = Format Into String(PIM_Data_Channels."IM%d Power 2" ("Enum")) -> (resulting string=w470:string)  [unwired: 3 in, 1 out]
            n219 = Add(x=w482, y=w481) -> (x+y=w475:i32)
            n220 = call "PIM Base Order to IM Order.vi"("Base Order (0)"=w475) -> ("IM Order"=w468:u8)  [unwired: 5 out]
            n221 = Index Array(array=w472, index=w481) -> (element=w476:dbl)
            n222 = Format Into String(format string=w470, w468) -> (resulting string=w469:string)  [unwired: 2 in, 1 out]
            n223 = Unbundle By Name(w483) -> ("Y"=w479:dbl[])
            n224 = Build Array (concatenate)(w479, w476) -> (w478:dbl[])
            n225 = Bundle By Name(cluster=w483, "Y"=w478) -> (w477:waveform(dbl))
            n226 = Set Waveform Attribute(5:w469, 6:w485, 7:w477) -> (3:w484:waveform(dbl))  [unwired: 1 in, 2 out]
            n227 = Format Into String(enum16{"dBm", "dBc"}."dBc" ("Measure.Ref Units")) -> (resulting string=w474:string)  [unwired: 3 in, 1 out]
          }
          frame Default {
            # "This property is not supported, we should\nNEVER reach this case."
            n228 = Delete From Array(array=w488, index=w489) -> (array with subset deleted=w487:waveform(dbl)[])  [unwired: 1 in, 1 out]
          }
        }
        n229 = Set Waveform Attribute(5:w41, 6:w42, 7:w43) -> (3:w44:waveform(dbl))  [unwired: 1 in, 2 out]
        n230 = Replace Array Subset(array=w46, new element=w44, index=w53) -> (w54:waveform(dbl)[])
      }
      n231 = Select(t=w35, s="Increment Cycles?", f=w36) -> (s? t:f=w34:i32)
      n232 = Bundle By Name(cluster=w38, "Measurement Cycles"=w34, "Data"=w24) -> (w37:T11)
    }
    frame True {
    }
  }
  "Updated Test Results" <- w2
